vi "Check Windows Platform.vi"(8 "Error In":errorcluster) -> (0 "Error Out":errorcluster)   [LabVIEW 2019, in "SLL Environment Variable.lvlib"]
doc: "Check if platform is Windows and generate a custom error for other platforms."
uses:
  <vilib>/SLL Toolkit/SLL Environment Variable/SLL Environment Variable.lvlib
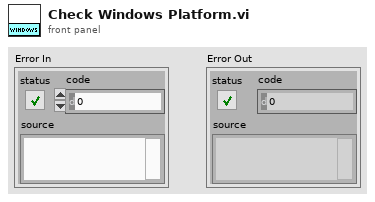
[diagram p1: front panel]
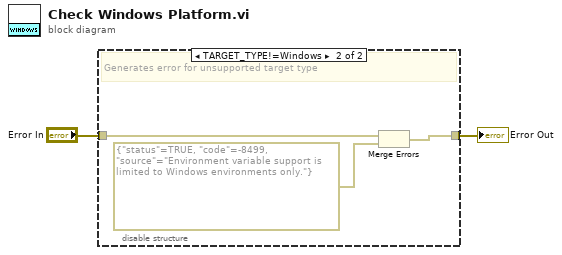
[diagram p0: block diagram]
diagram:
  n1 = disable-structure shown="TARGET_TYPE!=Windows" {
    disable-tunnel: "Error In" -> [w3 w6]
    disable-tunnel: [w3 w4] -> w1
    frame condition #0 (active) {
    }
    frame condition #1 {
      # "Generates error for unsupported target type"
      n2 = Merge Errors(w6, errorcluster {"status"=TRUE, "code"=-8499, "source"="Environment variable support is limited to Windows environments only."} ("Error In")) -> (w4:errorcluster)
    }
  }
  "Error Out" <- w1
